vi "MH_ChannelInitDone.vi"(8 "error in (no error)":errorcluster, 11 "SinglePhotonInterferenceUI in":refnum<class "SinglePhotonInterferenceUI.lvclass">) -> (0 "error out":errorcluster, 3 "SinglePhotonInterferenceUI out":refnum<class "SinglePhotonInterferenceUI.lvclass">)   [LabVIEW 2023, in "SinglePhotonInterferenceUI.lvlib" / "SinglePhotonInterferenceUI.lvclass"]
uses:
  SinglePhotonInterferenceUI.lvclass
  SinglePhotonInterferenceUI.lvclass/SinglePhotonInterferenceUI.ctl
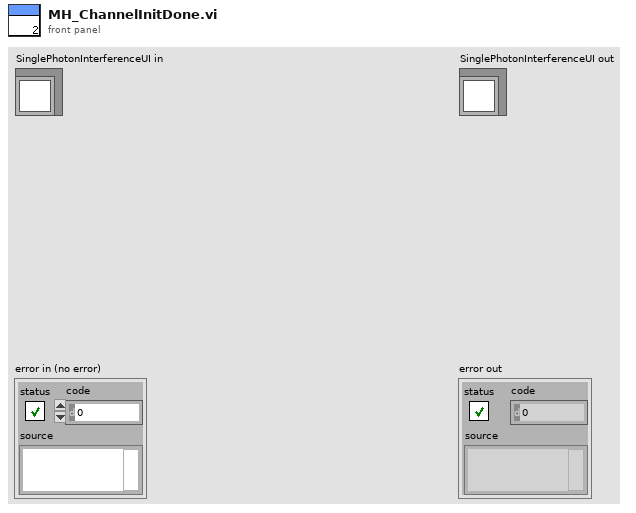
[diagram p1: front panel]
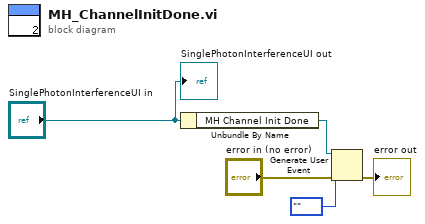
[diagram p0: block diagram]
diagram:
  n1 = Unbundle By Name("SinglePhotonInterferenceUI in") -> ("MH Channel Init Done"=w5:refnum<user-event>)
  n2 = Generate User Event(user event=w5, event data cluster=enum16{""}."" ("event data"), error in="error in (no error)") -> (error out=→"error out":errorcluster)  [unwired: 1 in, 1 out]
  "SinglePhotonInterferenceUI out" <- "SinglePhotonInterferenceUI in"
